vi "ToolStrip.vi"(5 "DropDownDirection":i32(ring)=7 items=["AboveLeft"=0, "AboveRight"=1, "BelowLeft"=2, "BelowRight"=3, "Left"=4, "Right"=5, "Default"=7], 6 "LayoutStyle":i32(ring) items=["StackWithOverflow", "HorizontalStackWithOverflow", "VerticalStackWithOverflow", "Flow", "Table"], 7 "TextDirection":i32(ring)=1 items=["Inherit", "Horizontal", "Vertical90", "Vertical270"], 10 "error in (no error)":errorcluster, 11 "ToolStrip":refnum<k24>) -> (2 "error out":errorcluster, 3 "ToolStrip out":refnum<class "MGI_ToolStrip.lvclass">)   [LabVIEW 2019, in "MGI_ToolStrip.lvclass"]
uses:
  MGI_ToolStrip.lvclass
  System.Windows.Forms
  MGI_ToolStrip.lvclass/MGI_ToolStrip.ctl
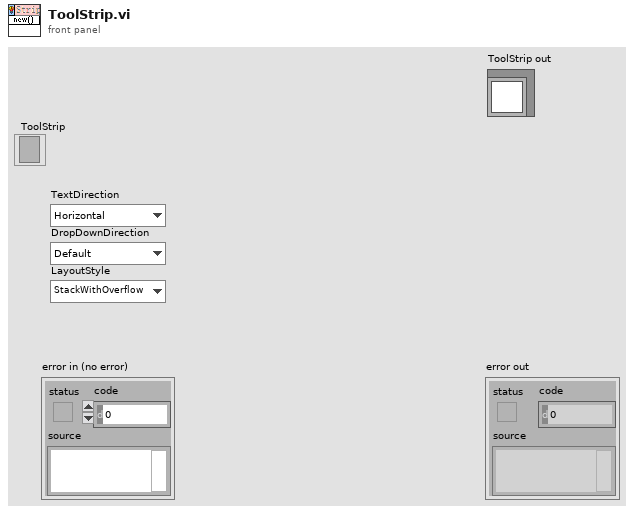
[diagram p1: front panel]
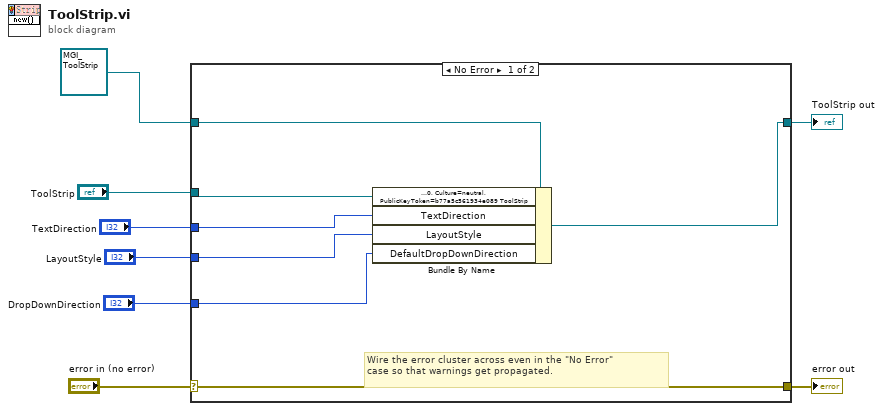
[diagram p0: block diagram]
diagram:
  n1 = case shown="No Error" "error in (no error)" {
    selector: "error in (no error)" -> [w15 w17]
    tunnel: [w15 w17] -> w7
    tunnel: [w12 w16] -> w5
    tunnel: refnum<class "MGI_ToolStrip.lvclass"> refnum ("ToolStrip in") -> [w14 w16]
    tunnel: "ToolStrip" -> [w13 _]
    tunnel: "TextDirection" -> [w11 _]
    tunnel: "LayoutStyle" -> [w10 _]
    tunnel: "DropDownDirection" -> [w9 _]
    frame No Error {
      # "Wire the error cluster across even in the \"No Error\"\ncase so that warnings get propagated."
      n2 = Bundle By Name(cluster=w14, "ToolStrip"=w13, "TextDirection"=w11, "LayoutStyle"=w10, "DefaultDropDownDirection"=w9) -> (w12:refnum<class "MGI_ToolStrip.lvclass">)
    }
    frame Error {
    }
  }
  "error out" <- w7
  "ToolStrip out" <- w5
